vi "ReadDate.vi"(8 "错误输入（无错误）":errorcluster caption="18000ERRIN", 11 "18000IN":refnum<k5>) -> (1 "18000OUT":dbl[](array[numeric]), 2 "18000ERROUT":errorcluster, 3 "18000TCPOUT":refnum<k5>)   [LabVIEW 2014]
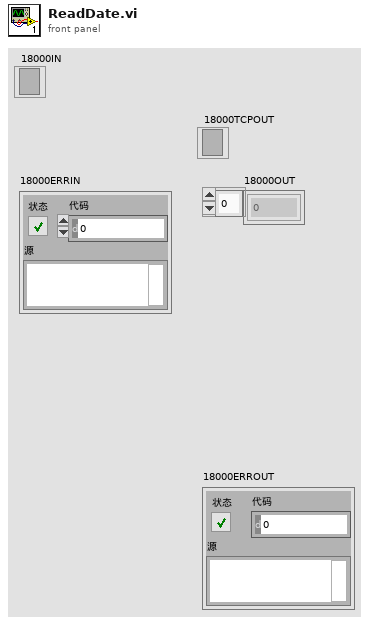
[diagram p1: front panel]
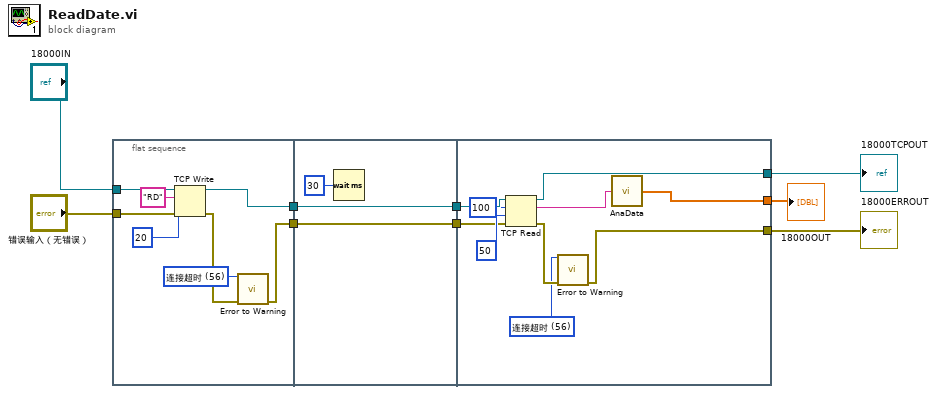
[diagram p0: block diagram]
diagram:
  n1 = flat-sequence {
    tunnel: "18000IN" -> [w16]
    tunnel: [w15] -> w9
    tunnel: "错误输入（无错误）" -> [w14]
    tunnel: [w10] -> w8
    tunnel: w9 -> [w19]
    tunnel: [w19] -> w7
    tunnel: [w18] -> w6
    tunnel: w8 -> [w18]
    tunnel: w7 -> [w30]
    tunnel: [w27] -> w2
    tunnel: w6 -> [w26]
    tunnel: [w22] -> w4
    tunnel: [w24] -> w5
    frame #0 {
      w11 = 56 items=["无错误", "参数错误", "内存已满", "超出区域", "文件结束", "文件已打开", "一般文件IO错误", "未找到文件", "文件权限错误", "磁盘已满", "路径副本", "打开过多文件", "未启用", "未找到资源文件", "无法添加资源", "未找到资源", "未找到图像", "图像内存错误", "画笔不存在", "配置错误类型", "配置未找到解析段", "配置解析错误", "配置内存错误", "错误外部代码格式", "错误外部代码偏移量", "外部代码不存在", "空窗口", "销毁窗口错误", "空菜单", "打印已中止", "错误打印记录", "打印驱动程序错误", "打印时窗口错误", "打印时内存错误", "打印对话框错误", "一般打印错误", "无效设备引用句柄", "设备未找到", "设备参数错误", "设备单位错误", "无法打开设备", "设备调用已中止", "一般错误", "用户已取消", "对象ID过低", "对象ID过高", "对象不在堆中", "未知的堆", "错误DefProc ID", "DefProc不在表格中", "范围外信息", "空方法", "未知信息", "不支持管理器调用", "错误地址", "连接过程中", "连接超时", "连接过程中", "不支持网络属性", "网络错误", "正在使用的地址", "系统缺少内存", "连接已中止", "连接已拒绝", "连接未建立", "连接已建立", "连接已关闭", "初始化错误（交互应用程序管理器）", "错误事件发生", "等待无约束事件发生处理程序", "事件发生队列溢出", "错误路径", "未发出信号量", "未识别类型（交互应用程序管理器）"] ("1st Error to Convert")
      n2 = TCP Write(connection ID=w16, data in="RD" ("数据输入"), error in (no error)=w14, 9:20 ("超时毫秒(25000)")) -> (connection ID out=w15:refnum<k5>, error out=w12:errorcluster)  [unwired: 1 out]
      n3 = call <vilib>:"Error to Warning.vi"("1st Error to Convert"=w11, "error in"=w12) -> ("warning out"=w10:errorcluster)  [unwired: 13 in]
    }
    frame #1 {
      n4 = Wait (ms)(milliseconds to wait=u32 30 ("等待时间（毫秒）")) -> ()  [unwired: 1 out]
    }
    frame #2 {
      w21 = 56 items=["无错误", "参数错误", "内存已满", "超出区域", "文件结束", "文件已打开", "一般文件IO错误", "未找到文件", "文件权限错误", "磁盘已满", "路径副本", "打开过多文件", "未启用", "未找到资源文件", "无法添加资源", "未找到资源", "未找到图像", "图像内存错误", "画笔不存在", "配置错误类型", "配置未找到解析段", "配置解析错误", "配置内存错误", "错误外部代码格式", "错误外部代码偏移量", "外部代码不存在", "空窗口", "销毁窗口错误", "空菜单", "打印已中止", "错误打印记录", "打印驱动程序错误", "打印时窗口错误", "打印时内存错误", "打印对话框错误", "一般打印错误", "无效设备引用句柄", "设备未找到", "设备参数错误", "设备单位错误", "无法打开设备", "设备调用已中止", "一般错误", "用户已取消", "对象ID过低", "对象ID过高", "对象不在堆中", "未知的堆", "错误DefProc ID", "DefProc不在表格中", "范围外信息", "空方法", "未知信息", "不支持管理器调用", "错误地址", "连接过程中", "连接超时", "连接过程中", "不支持网络属性", "网络错误", "正在使用的地址", "系统缺少内存", "连接已中止", "连接已拒绝", "连接未建立", "连接已建立", "连接已关闭", "初始化错误（交互应用程序管理器）", "错误事件发生", "等待无约束事件发生处理程序", "事件发生队列溢出", "错误路径", "未发出信号量", "未识别类型（交互应用程序管理器）"] ("1st Error to Convert")
      n5 = TCP Read(connection ID=w30, bytes to read=100 ("读取的字节"), error in (no error)=w26, 9:50 ("超时毫秒(25000)")) -> (connection ID out=w27:refnum<k5>, data out=w25:string, error out=w23:errorcluster)  [unwired: 1 in]
      n6 = call <vilib>:"Error to Warning.vi"("1st Error to Convert"=w21, "error in"=w23) -> ("warning out"=w22:errorcluster)  [unwired: 13 in]
      n7 = call "AnaData.vi"("字符串"=w25) -> ("数组"=w24:dbl[])
    }
  }
  "18000OUT" <- w5
  "18000ERROUT" <- w4
  "18000TCPOUT" <- w2
